vi "SetExposure.vi"(8 "error in (no error)":errorcluster, 10 "Arg":string, 11 "PCO in":refnum<class "PCO_Camera.lvclass">) -> (0 "error out":errorcluster, 2 "setValue out":dbl, 3 "PCO out":refnum<class "PCO_Camera.lvclass">)   [LabVIEW 2020, in "PCO_Camera.lvclass"]
uses:
  PCO_Camera.lvclass
  PCO_Camera.lvclass/PCO_Camera.ctl
  pco.labview/pco.camera/Camera.lvclass
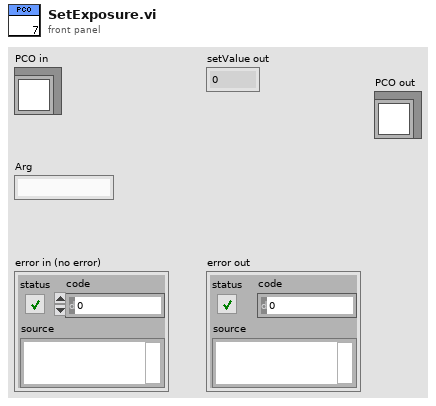
[diagram p1: front panel]
types:
  T1 = enum16{"sequence", "sequence non blocking", "ring buffer", "fifo", "sequence_dpcore", "sequence_non_blocking_dpcore", "ring_buffer_dpcore", "fifo_dpcore", "tif", "multitif", "pcoraw", "b16", "dicom", "multidicom"}
  T2 = typedef "Camera.lvclass/binning.ctl" = cluster{"vert":u16, "horz":u16}
  T3 = cluster{"exposure_time_s":dbl, "delay_time_s":dbl, "roi":cluster{"x0":u64, "y0":u64, "x1":u64, "y1":u64}, "timestamp_mode":u16, "pixelrate":u32, "trigger_mode":u16, "acquire_mode":u16, "metadata_mode":u16, "noisefilter_mode":u16, "binning":T2}
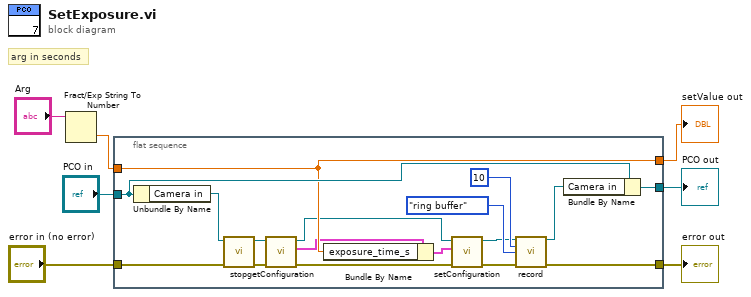
[diagram p0: block diagram]
diagram:
  # "arg in seconds"
  n1 = Fract/Exp String To Number(string="Arg") -> (number=w3:dbl)  [unwired: 3 in, 1 out]
  n2 = flat-sequence {
    tunnel: "PCO in" -> [w24]
    tunnel: [w22] -> w5
    tunnel: "error in (no error)" -> [w15]
    tunnel: w3 -> [w23]
    tunnel: [w23] -> w2
    tunnel: [w8] -> w1
    frame #0 {
      n3 = Unbundle By Name(w24) -> ("Camera in"=w16:refnum<class "Camera.lvclass">)
      n4 = call-dynamic "stop.vi"("error in (no error)"=w15, "Camera in"=w16) -> ("error out"=w14:errorcluster, "Camera out"=w17:refnum<class "Camera.lvclass">)  [unwired: 8 in]
      n5 = call-dynamic "getConfiguration.vi"("error in (no error)"=w14, "Camera in"=w17) -> ("error out"=w21:errorcluster, "configuration"=w19:T3, "Camera out"=w20:refnum<class "Camera.lvclass">)  [unwired: 7 in]
      n6 = Bundle By Name(cluster=w19, "exposure_time_s"=w23) -> (w18:T3)
      n7 = call-dynamic "setConfiguration.vi"("error in (no error)"=w21, "configuration"=w18, "Camera in"=w20) -> ("error out"=w9:errorcluster, "Camera out"=w11:refnum<class "Camera.lvclass">)  [unwired: 7 in]
      n8 = call-dynamic "record.vi"("Camera in"=w11, "num_images"=u32 10, "record_mode"=T1."ring buffer", "error in (no error)"=w9) -> ("Camera out"=w10:refnum<class "Camera.lvclass">, "error out"=w8:errorcluster)  [unwired: 10 in]
      n9 = Bundle By Name(cluster=w24, "Camera in"=w10) -> (w22:refnum<class "PCO_Camera.lvclass">)
    }
  }
  "error out" <- w1
  "PCO out" <- w5
  "setValue out" <- w2
